vi "Get Payload DVR.vi"(7 "Msg":refnum<class "Msg.lvclass">) -> (3 "Payload DVR":refnum<data-value>)   [LabVIEW 2020, in "_Template.lvlib" / "{{Msg}}.lvlib" / "Msg.lvclass"]
uses:
  Msg.lvclass
  Msg.lvclass/Msg.ctl
  Payload.ctl
  {{Msg}}.lvlib
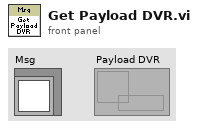
[diagram p1: front panel]
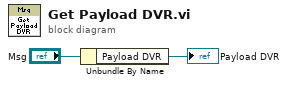
[diagram p0: block diagram]
diagram:
  n1 = Unbundle By Name("Msg") -> ("Payload DVR"=→"Payload DVR":refnum<data-value>)
